vi "Time_diff.vi"(9 "End_Time":string, 11 "Start_Time":string) -> (2 "Time_diff":string)   [LabVIEW 2014]
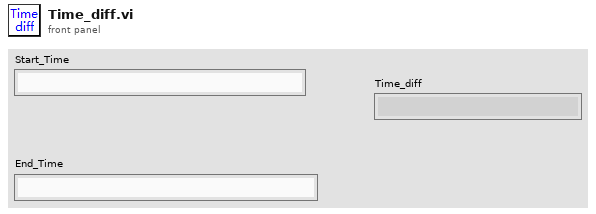
[diagram p1: front panel]
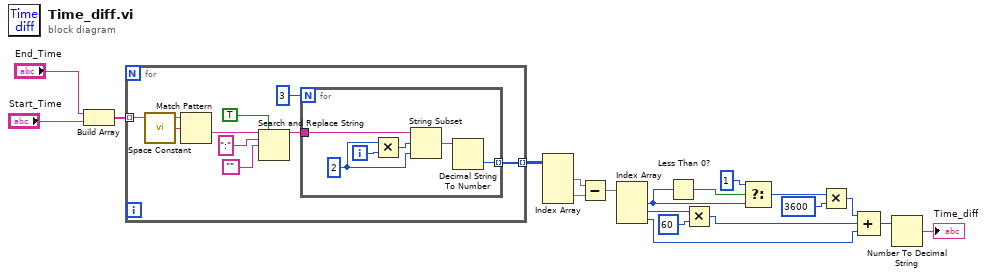
[diagram p0: block diagram]
diagram:
  n1 = Build Array("End_Time", "Start_Time") -> (w17:string[])
  n2 = for {
    tunnel: w17 -> [w21] mode=indexing
    tunnel: [w20] -> w16 mode=indexing
    n3 = call <vilib>:"Space Constant.vi"() -> ("String"=w27:string)
    n4 = Match Pattern(string=w21, regular expression=w27) -> (after substring=w26:string)  [unwired: 1 in, 3 out]
    n5 = Search and Replace String(replace all?=TRUE ("replace all? (F)"), input string=w26, search string=":", replace string="") -> (result string=w23:string)  [unwired: 4 in, 3 out]
    n6 = for {
      N: 3 -> [_]
      tunnel: w23 -> [w34]
      tunnel: [w29] -> w20 mode=indexing
      i -> [w33]
      w31 = 2 ("x")
      n7 = Multiply(x=w31, y=w33) -> (x*y=w32:i32)
      n8 = String Subset(string=w34, offset (0)=w32, length (rest)=w31) -> (substring=w30:string)
      n9 = Decimal String To Number(string=w30) -> (number=w29:i32)  [unwired: 2 in, 1 out]
    }
  }
  n10 = Index Array(array=w16) -> (element #1=w15:i32[], element #2=w14:i32[])  [unwired: 4 in]
  n11 = Subtract(x=w15, y=w14) -> (x-y=w13:i32[])
  n12 = Index Array(array=w13) -> (element #1=w3:i32, element #2=w11:i32, element #3=w7:i32)  [unwired: 3 in]
  n13 = Less Than 0?(x=w3) -> (x < 0?=w5:bool)
  n14 = Multiply(x=w11, y=60) -> (x*y=w8:i32)
  n15 = Select(t=1 ("y"), s=w5, f=w3) -> (s? t:f=w2:i32)
  n16 = Multiply(x=w2, y=3600) -> (x*y=w9:i32)
  n17 = Compound Arithmetic op=ADD(w9, w8, w7) -> (w1:i32)
  n18 = Number To Decimal String(number=w1) -> (decimal integer string=→"Time_diff":string)  [unwired: 1 in]
